vi "UPDATE USER CLUSTER.vi"(10 "REFERENCES":T2, 11 "USER INFO IN":T1) -> (2 "DO NOT PROCEED?":bool, 3 "USER INFO OUT":T1)   [LabVIEW 2019]
uses:
  Controls/References Cluster.ctl
  Controls/Custom Calendar/Custom Calendar.xctl
  <vilib>/regexp/Match Regular Expression.xnode
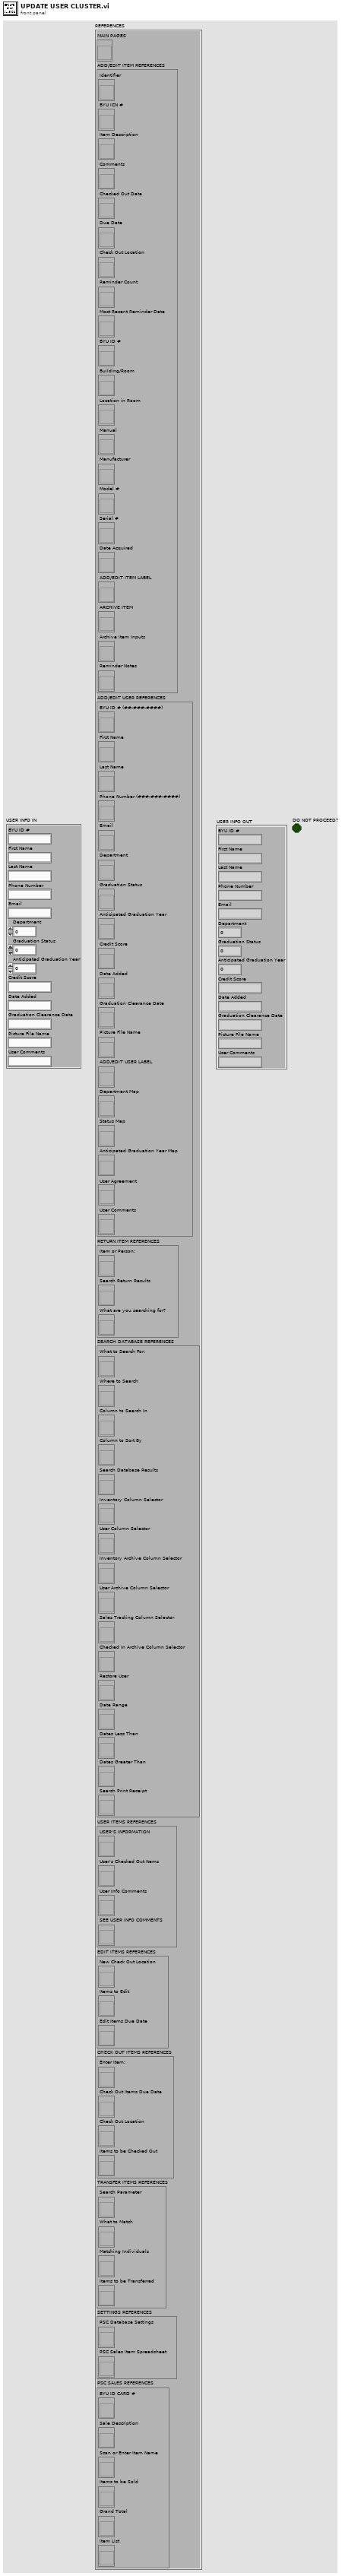
[diagram p1: front panel]
types:
  T1 = cluster{"BYU ID #":string, "First Name":string, "Last Name":string, "Phone Number":string, "Email":string, "Department":u16, "Graduation Status":u16, "Anticipated Graduation Year":u16, "Credit Score":string, "Date Added":string, "Graduation Clearance Date":string, "Picture File Name":string, "User Comments":string}
  T2 = typedef "References Cluster.ctl" = cluster{"MAIN PAGES":refnum<vi>, "ADD/EDIT ITEM REFERENCES":cluster{"Identifier":refnum<vi>, "BYU ICN #":refnum<vi>, "Item Description":refnum<vi>, "Comments":refnum<vi>, "Checked Out Date":refnum<vi>, "Due Date":refnum<vi>, "Check Out Location":refnum<vi>, "Reminder Count":refnum<vi>, "Most Recent Reminder Date":refnum<vi>, "BYU ID #":refnum<vi>, "Building/Room":refnum<vi>, "Location in Room":refnum<vi>, "Manual":refnum<vi>, "Manufacturer":refnum<vi>, "Model #":refnum<vi>, "Serial #":refnum<vi>, "Date Acquired":refnum<vi>, "ADD/EDIT ITEM LABEL":refnum<vi>, "ARCHIVE ITEM":refnum<vi>, "Archive Item Inputs":refnum<vi>, "Reminder Notes":refnum<vi>}, "ADD/EDIT USER REFERENCES":cluster{"BYU ID # (##-###-####)":refnum<vi>, "First Name":refnum<vi>, "Last Name":refnum<vi>, "Phone Number (###-###-####)":refnum<vi>, "Email":refnum<vi>, "Department":refnum<vi>, "Graduation Status":refnum<vi>, "Anticipated Graduation Year":refnum<vi>, "Credit Score":refnum<vi>, "Date Added":refnum<vi>, "Graduation Clearance Date":refnum<vi>, "Picture File Name":refnum<vi>, "ADD/EDIT USER LABEL":refnum<vi>, "Department Map":refnum<vi>, "Status Map":refnum<vi>, "Anticipated Graduation Year Map":refnum<vi>, "User Agreement":refnum<vi>, "User Comments":refnum<vi>}, "RETURN ITEM REFERENCES":cluster{"Item or Person:":refnum<vi>, "Search Return Results":refnum<vi>, "What are you searching for?":refnum<vi>}, "SEARCH DATABASE REFERENCES":cluster{"What to Search For:":refnum<vi>, "Where to Search":refnum<vi>, "Column to Search In":refnum<vi>, "Column to Sort By":refnum<vi>, "Search Database Results":refnum<vi>, "Inventory Column Selector":refnum<vi>, "User Column Selector":refnum<vi>, "Inventory Archive Column Selector":refnum<vi>, "User Archive Column Selector":refnum<vi>, "Sales Tracking Column Selector":refnum<vi>, "Checked In Archive Column Selector":refnum<vi>, "Restore User":refnum<vi>, "Date Range":refnum<vi>, "Dates Less Than":refnum<vi>, "Dates Greater Than":refnum<vi>, "Search Print Receipt":refnum<vi>}, "USER ITEMS REFERENCES":cluster{"USER'S INFORMATION":refnum<vi>, "User's Checked Out Items":refnum<vi>, "User Info Comments":refnum<vi>, "SEE USER INFO COMMENTS":refnum<vi>}, "EDIT ITEMS REFERENCES":cluster{"New Check Out Location":refnum<vi>, "Items to Edit":refnum<vi>, "Edit Items Due Date":refnum<vi>}, "CHECK OUT ITEMS REFERENCES":cluster{"Enter Item:":refnum<vi>, "Check Out Items Due Date":refnum<vi>, "Check Out Location":refnum<vi>, "Items to be Checked Out":refnum<vi>}, "TRANSFER ITEMS REFERENCES":cluster{"Search Parameter":refnum<vi>, "What to Match":refnum<vi>, "Matching Individuals":refnum<vi>, "Items to be Transferred":refnum<vi>}, "SETTINGS REFERENCES":cluster{"PSC Database Settings":refnum<vi>, "PSC Sales Item Spreadsheet":refnum<vi>}, "PSC SALES REFERENCES":cluster{"BYU ID CARD #":refnum<vi>, "Sale Description":refnum<vi>, "Scan or Enter Item Name":refnum<vi>, "Items to be Sold":refnum<vi>, "Grand Total":refnum<vi>, "Item List":refnum<vi>}}
  T3 = cluster{"BYU ID # (##-###-####)":refnum<vi>, "First Name":refnum<vi>, "Last Name":refnum<vi>, "Phone Number (###-###-####)":refnum<vi>, "Email":refnum<vi>, "Department":refnum<vi>, "Graduation Status":refnum<vi>, "Anticipated Graduation Year":refnum<vi>, "Credit Score":refnum<vi>, "Date Added":refnum<vi>, "Graduation Clearance Date":refnum<vi>, "Picture File Name":refnum<vi>, "ADD/EDIT USER LABEL":refnum<vi>, "Department Map":refnum<vi>, "Status Map":refnum<vi>, "Anticipated Graduation Year Map":refnum<vi>, "User Agreement":refnum<vi>, "User Comments":refnum<vi>}
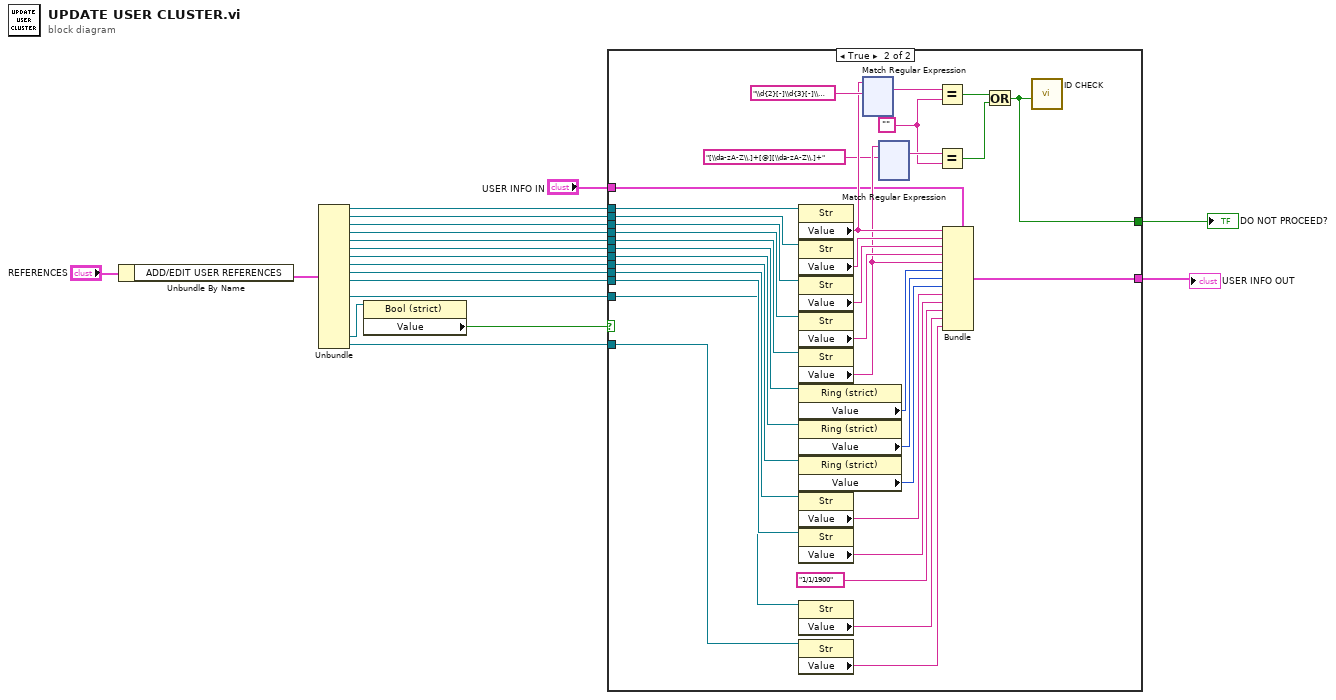
[diagram p0: block diagram]
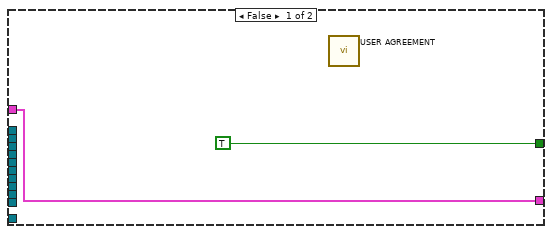
[diagram p2: hidden frame]
diagram:
  n1 = Unbundle By Name("REFERENCES") -> ("ADD/EDIT USER REFERENCES"=w8:T3)
  n2 = Unbundle(w8) -> ("BYU ID # (##-###-####)"=w19:refnum<vi>, "First Name"=w18:refnum<vi>, "Last Name"=w9:refnum<vi>, "Phone Number (###-###-####)"=w17:refnum<vi>, "Email"=w16:refnum<vi>, "Department"=w15:refnum<vi>, "Graduation Status"=w10:refnum<vi>, "Anticipated Graduation Year"=w14:refnum<vi>, "Credit Score"=w13:refnum<vi>, "Date Added"=w12:refnum<vi>, "Picture File Name"=w11:refnum<vi>, "User Agreement"=w6:refnum<vi>, "User Comments"=w1:refnum<vi>)  [unwired: 5 out]
  n3 = property class="Bool (strict)"(reference=w6) -> ("Value"=w5:bool)  [unwired: 1 in, 2 out]
  n4 = case shown="True" w5 {
    tunnel: w19 -> [_ w56]
    tunnel: w18 -> [_ w55]
    tunnel: w17 -> [_ w54]
    tunnel: w16 -> [_ w53]
    tunnel: w15 -> [_ w52]
    tunnel: w14 -> [_ w51]
    tunnel: w13 -> [_ w50]
    tunnel: w12 -> [_ w49]
    tunnel: w11 -> [_ w48]
    tunnel: w10 -> [_ w47]
    tunnel: w9 -> [_ w46]
    tunnel: [TRUE w26] -> w4
    tunnel: [w20 w25] -> w3
    tunnel: "USER INFO IN" -> [w20 w24]
    tunnel: w1 -> [_ w23]
    frame False {
      n5 = call "USER AGREEMENT"() -> ()  [unwired: 10 in, 2 out]
    }
    frame True {
      w29 = ""
      n6 = property class="Str"(reference=w56) -> ("Value"=w33:string)  [unwired: 1 in, 2 out]
      n7 = property class="Str"(reference=w55) -> ("Value"=w45:string)  [unwired: 1 in, 2 out]
      n8 = property class="Str"(reference=w46) -> ("Value"=w44:string)  [unwired: 1 in, 2 out]
      n9 = property class="Str"(reference=w54) -> ("Value"=w43:string)  [unwired: 1 in, 2 out]
      n10 = property class="Str"(reference=w53) -> ("Value"=w32:string)  [unwired: 1 in, 2 out]
      n11 = property class="Ring (strict)"(reference=w52) -> ("Value"=w42:u16)  [unwired: 1 in, 2 out]
      n12 = property class="Ring (strict)"(reference=w47) -> ("Value"=w41:u16)  [unwired: 1 in, 2 out]
      n13 = property class="Ring (strict)"(reference=w51) -> ("Value"=w40:u16)  [unwired: 1 in, 2 out]
      n14 = property class="Str"(reference=w50) -> ("Value"=w39:string)  [unwired: 1 in, 2 out]
      n15 = property class="Str"(reference=w49) -> ("Value"=w38:string)  [unwired: 1 in, 2 out]
      n16 = property class="Str"(reference=w48) -> ("Value"=w37:string)  [unwired: 1 in, 2 out]
      n17 = property class="Str"(reference=w23) -> ("Value"=w22:string)  [unwired: 1 in, 2 out]
      n18 = xnode "Match Regular Expression"("input string"=w33, "regular expression"="\\d{2}[-]\\d{3}[-]\\d{4}") -> ("whole match"=w35:string)  [unwired: 4 in, 4 out]
      n19 = xnode "Match Regular Expression"("input string"=w32, "regular expression"="[\\da-zA-Z\\.]+[@][\\da-zA-Z\\.]+" ("search string")) -> ("whole match"=w30:string)  [unwired: 4 in, 4 out]
      n20 = Equal?(x=w35, y=w29) -> (x = y?=w28:bool)
      n21 = Equal?(x=w30, y=w29) -> (x = y?=w27:bool)
      n22 = Bundle(cluster=w24, "BYU ID #"=w33, "First Name"=w45, "Last Name"=w44, "Phone Number"=w43, "Email"=w32, "Department"=w42, "Graduation Status"=w41, "Anticipated Graduation Year"=w40, "Credit Score"=w39, "Date Added"=w38, "Graduation Clearance Date"="1/1/1900", "Picture File Name"=w37, "User Comments"=w22) -> (w25:T1)
      n23 = Or(x=w28, y=w27) -> (x .or. y?=w26:bool)
      n24 = call "ID CHECK"("Enable"=w26) -> ()  [unwired: 9 in, 2 out]
    }
  }
  "DO NOT PROCEED?" <- w4
  "USER INFO OUT" <- w3
